vi "Generate Trajectory for Alignment.vi"(8 "Setpoints":T1={"x setpoint"=-0.39, "y setpoint"=-0.8, "th setpoint"=0.0}, 9 "th":dbl=5.222202292601764, 10 "y":dbl=-5.250819805384862, 11 "x":dbl=0.8562227067038787) -> (2 "Updated Waypoints":cluster{"x":dbl, "y":dbl, "th":dbl}[](array[cluster]), 3 "Trajectory Data Out":T3(array[cluster])=[{"Segment Name"="Linear 0", "Type"=enum."Accel Straight", "Traj Pos Points"=[{"x"=0.8100058273974486, "y"=-3.967975741983552, "th"=5.222202301025391}, {"x"=0.7603878706355013, "y"=-3.830783760791278, "th"=5.0782023010253905}, {"x"=0.7073688364180365, "y"=-3.68418791485404, "th"=4.877149425506592}, {"x"=0.6509487247450543, "y"=-3.5281882041718386, "th"=4.676096549987793}, {"x"=0.5911275356165546, "y"=-3.3627846287446737, "th"=4.475043674468994}, {"x"=0.5279052690325376, "y"=-3.1879771885725448, "th"=4.273990798950195}, {"x"=0.46128192499300325, "y"=-3.0037658836554524, "th"=4.072937923431397}, {"x"=0.39465858095346884, "y"=-2.8195545787383596, "th"=3.8718850479125977}, {"x"=0.32803523691393444, "y"=-2.6353432738212668, "th"=3.6708321723937987}, {"x"=0.26141189287440003, "y"=-2.451131968904174, "th"=3.469779296875}, {"x"=0.198189626290383, "y"=-2.276324528732045, "th"=3.2687264213562015}, {"x"=0.1383684371618834, "y"=-2.1109209533048796, "th"=3.0676735458374025}, {"x"=0.0819483254889012, "y"=-1.954921242622678, "th"=2.8666206703186035}, {"x"=0.02892929127143639, "y"=-1.8083253966854402, "th"=2.6655677947998044}, {"x"=-0.020688665490511016, "y"=-1.671133415493166, "th"=2.4645149192810054}, {"x"=-0.06690554479694102, "y"=-1.5433452990458556, "th"=2.2634620437622064}, {"x"=-0.10972134664785363, "y"=-1.4249610473435088, "th"=2.0624091682434074}, {"x"=-0.14913607104324883, "y"=-1.315980660386126, "th"=1.8613562927246083}, {"x"=-0.18514971798312663, "y"=-1.2164041381737067, "th"=1.6603034172058093}, {"x"=-0.21776228746748705, "y"=-1.1262314807062512, "th"=1.4592505416870103}, {"x"=-0.24697377949633004, "y"=-1.0454626879837594, "th"=1.2581976661682113}, {"x"=-0.27278419406965565, "y"=-0.9740977600062313, "th"=1.0571447906494127}, {"x"=-0.29519353118746383, "y"=-0.9121366967736668, "th"=0.8560919151306141}, {"x"=-0.31420179084975464, "y"=-0.8595794982860661, "th"=0.6550390396118155}, {"x"=-0.329808973056528, "y"=-0.816426164543429, "th"=0.45398616409301695}, {"x"=-0.342015077807784, "y"=-0.7826766955457557, "th"=0.2529332885742184}, {"x"=-0.35082010510352263, "y"=-0.7583310912930461, "th"=0.055585002899170455}, {"x"=-0.3562240549437438, "y"=-0.7433893517853002, "th"=0.002236717224122664}, {"x"=-0.35822692732844763, "y"=-0.737851477022518, "th"=0.002236717224122664}], "Traj Vel Points"=[{"V"=7.294446746788231, "Omega"=-0.0, "V vector"={"y"=-7.056933814139086, "x"=-1.8462498434907955}}, {"V"=7.794446746788231, "Omega"=-7.2, "V vector"={"y"=-7.535671418858484, "x"=-1.991747061129249}}, {"V"=8.294446746788232, "Omega"=-10.052643775939941, "V vector"={"y"=-8.011584634482254, "x"=-2.1476402119148625}}, {"V"=8.794446746788232, "Omega"=-10.052643775939941, "V vector"={"y"=-8.486490625788083, "x"=-2.306896278662117}}, {"V"=9.294446746788232, "Omega"=-10.052643775939941, "V vector"={"y"=-8.960371657345226, "x"=-2.4695100913190724}}, {"V"=9.794446746788232, "Omega"=-10.052643775939941, "V vector"={"y"=-9.433210017677535, "x"=-2.635476396794092}}, {"V"=9.794446746788232, "Omega"=-10.052643775939941, "V vector"={"y"=-9.423903981638178, "x"=-2.6685615639393947}}, {"V"=9.794446746788232, "Omega"=-10.052643775939941, "V vector"={"y"=-9.414481906133277, "x"=-2.701613872254829}}, {"V"=9.794446746788232, "Omega"=-10.052643775939941, "V vector"={"y"=-9.404943907179781, "x"=-2.7346329147570203}}, {"V"=9.294446746788232, "Omega"=-10.052643775939941, "V vector"={"y"=-8.91566678376851, "x"=-2.6263332099505634}}, {"V"=8.794446746788232, "Omega"=-10.052643775939941, "V vector"={"y"=-8.427271425386172, "x"=-2.5146351435076726}}, {"V"=8.294446746788232, "Omega"=-10.052643775939941, "V vector"={"y"=-7.939775651158667, "x"=-2.3995435908884546}}, {"V"=7.794446746788232, "Omega"=-10.052643775939941, "V vector"={"y"=-7.453197256780454, "x"=-2.2810635107418573}}, {"V"=7.294446746788232, "Omega"=-10.052643775939941, "V vector"={"y"=-6.967554014150215, "x"=-2.1591999448009993}}, {"V"=6.794446746788232, "Omega"=-10.052643775939941, "V vector"={"y"=-6.482863671006963, "x"=-2.0339580177769934}}, {"V"=6.294446746788232, "Omega"=-10.052643775939941, "V vector"={"y"=-5.99914395056661, "x"=-1.9053429372511914}}, {"V"=5.794446746788232, "Omega"=-10.052643775939941, "V vector"={"y"=-5.516412551158996, "x"=-1.7733599935659488}}, {"V"=5.294446746788232, "Omega"=-10.052643775939941, "V vector"={"y"=-5.034687145865371, "x"=-1.63801455971383}}, {"V"=4.794446746788232, "Omega"=-10.052643775939941, "V vector"={"y"=-4.553985382156366, "x"=-1.4993120912253046}}, {"V"=4.294446746788232, "Omega"=-10.052643775939941, "V vector"={"y"=-4.074324881530425, "x"=-1.3572581260549188}}, {"V"=3.794446746788232, "Omega"=-10.052643775939941, "V vector"={"y"=-3.595723239152738, "x"=-1.2118582844659433}}, {"V"=3.294446746788232, "Omega"=-10.052643775939941, "V vector"={"y"=-3.118198023494648, "x"=-1.0631182689134988}}, {"V"=2.794446746788232, "Omega"=-10.052643775939941, "V vector"={"y"=-2.641766775973572, "x"=-0.9110438639261721}}, {"V"=2.294446746788232, "Omega"=-10.052643775939941, "V vector"={"y"=-2.166447010593411, "x"=-0.7556409359861169}}, {"V"=1.794446746788232, "Omega"=-10.052643775939941, "V vector"={"y"=-1.692256213585474, "x"=-0.5969154334076338}}, {"V"=1.294446746788232, "Omega"=-10.052643775939941, "V vector"={"y"=-1.2192118430499221, "x"=-0.4348733862142511}}, {"V"=0.7944467467882319, "Omega"=-9.867414283752396, "V vector"={"y"=-0.7473487535270189, "x"=-0.26947258503234844}}, {"V"=0.2944467467882319, "Omega"=-2.6674142837523886, "V vector"={"y"=-0.2768976473427397, "x"=-0.1001328097589842}}, {"V"=0.0, "Omega"=-0.0, "V vector"={"y"=-0.0, "x"=-0.0}}], "Accel Index"=6, "Decel Index"=9}, {"Segment Name"="", "Type"=enum."Accel Straight", "Traj Pos Points"=[], "Traj Vel Points"=[], "Accel Index"=0, "Decel Index"=0}])   [LabVIEW 2023]
uses:
  bordeaux-pathinator/Bordeaux/Types/Segment Type.ctl
  bordeaux-pathinator/Bordeaux/Types/Angluar Limits.ctl
  bordeaux-pathinator/Bordeaux/Types/Drive Type.ctl
  bordeaux-pathinator/Bordeaux/Types/Limits.ctl
  Framework/Robot Global Data.vi
panel:
  in  "Ft per ft/sec":dbl=0.167
  out "Expected Distance":dbl=3.664199722009253
  out "Time & Dist":cluster{"Time (s)":dbl, "Distance (ft)":dbl}={"Time (s)"=0.58, "Distance (ft)"=3.664199722009253}
  out "past gen speed":u32=4
  out "Waveform Chart":dbl[](graph)=[7.294446746788231, 7.794446746788231, 8.294446746788232, 8.794446746788232, 9.294446746788232, 9.794446746788232, 9.794446746788232, 9.794446746788232, 9.794446746788232, 9.294446746788232, 8.794446746788232, 8.294446746788232, 7.794446746788232, 7.294446746788232, 6.794446746788232, 6.294446746788232, 5.794446746788232, 5.294446746788232, 4.794446746788232, 4.294446746788232, 3.794446746788232, 3.294446746788232, 2.794446746788232, 2.294446746788232, 1.794446746788232, 1.294446746788232, 0.7944467467882319, 0.2944467467882319, 0.0]
  out "Error":cluster{dbl, dbl, "th":dbl}={1.2462227067038787, -3.4457638584308623, "th"=5.222202292601764}
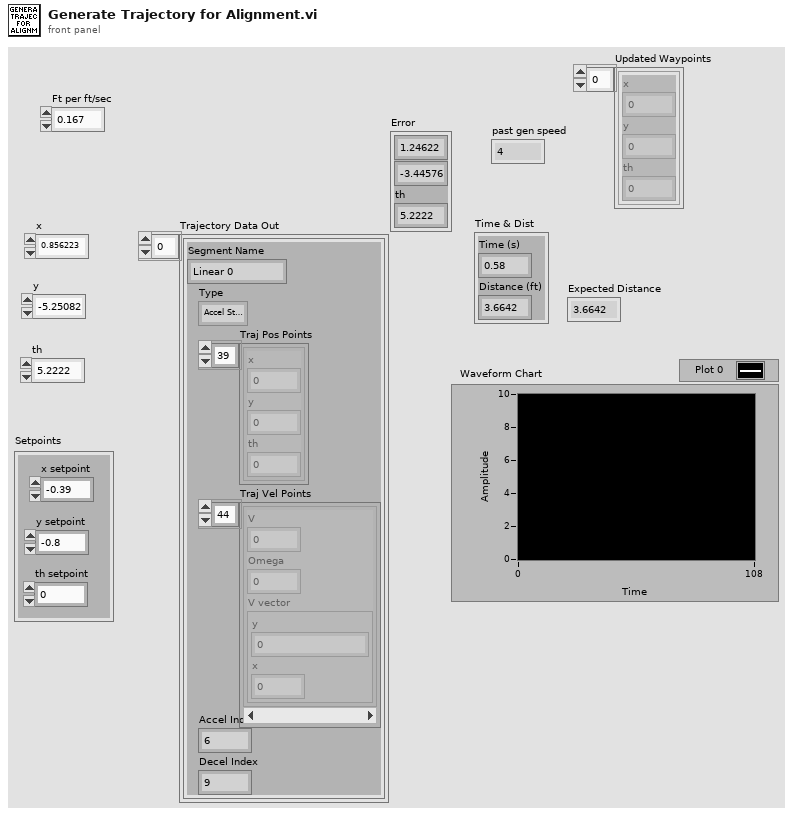
[diagram p1: front panel]
types:
  T1 = cluster{"x setpoint":dbl, "y setpoint":dbl, "th setpoint":dbl}
  T2 = typedef "Segment Type.ctl" = enum16{"Accel Straight", "Const Straight", "Blend", "Circle", "Bezier"}
  T3 = cluster{"Segment Name":string, "Type":T2, "Traj Pos Points":cluster{"x":dbl, "y":dbl, "th":dbl}[], "Traj Vel Points":cluster{"V":dbl, "Omega":dbl, "V vector":cluster{"y":dbl, "x":dbl}}[], "Accel Index":i32, "Decel Index":i32}[]
  T4 = typedef "Limits.ctl" = cluster{"Velocity (fps)":dbl, "Accel (fps^2)":dbl, "Jerk (fps^3)":dbl, "StoopidFast (fps)":dbl}
  T5 = typedef "Drive Type.ctl" = enum16{"Nonholonomic", "Holonomic"}
  T6 = typedef "Angluar Limits.ctl" = cluster{"Velocity (deg/s)":dbl, "Accel (deg/s^2)":dbl, "Jerk (deg/s^3)":dbl}
  T7 = typedef "Robot Velocities.ctl" = cluster{"X Velocity":dbl, "Y Velocity":dbl, "Rotational \nVelocity":dbl}
  T8 = cluster{"x setpoint":dbl, "y setpoint":dbl, "th setpoint":dbl}[]
  T9 = cluster{"V":dbl, "Omega":dbl, "V vector":cluster{"y":dbl, "x":dbl}}[]
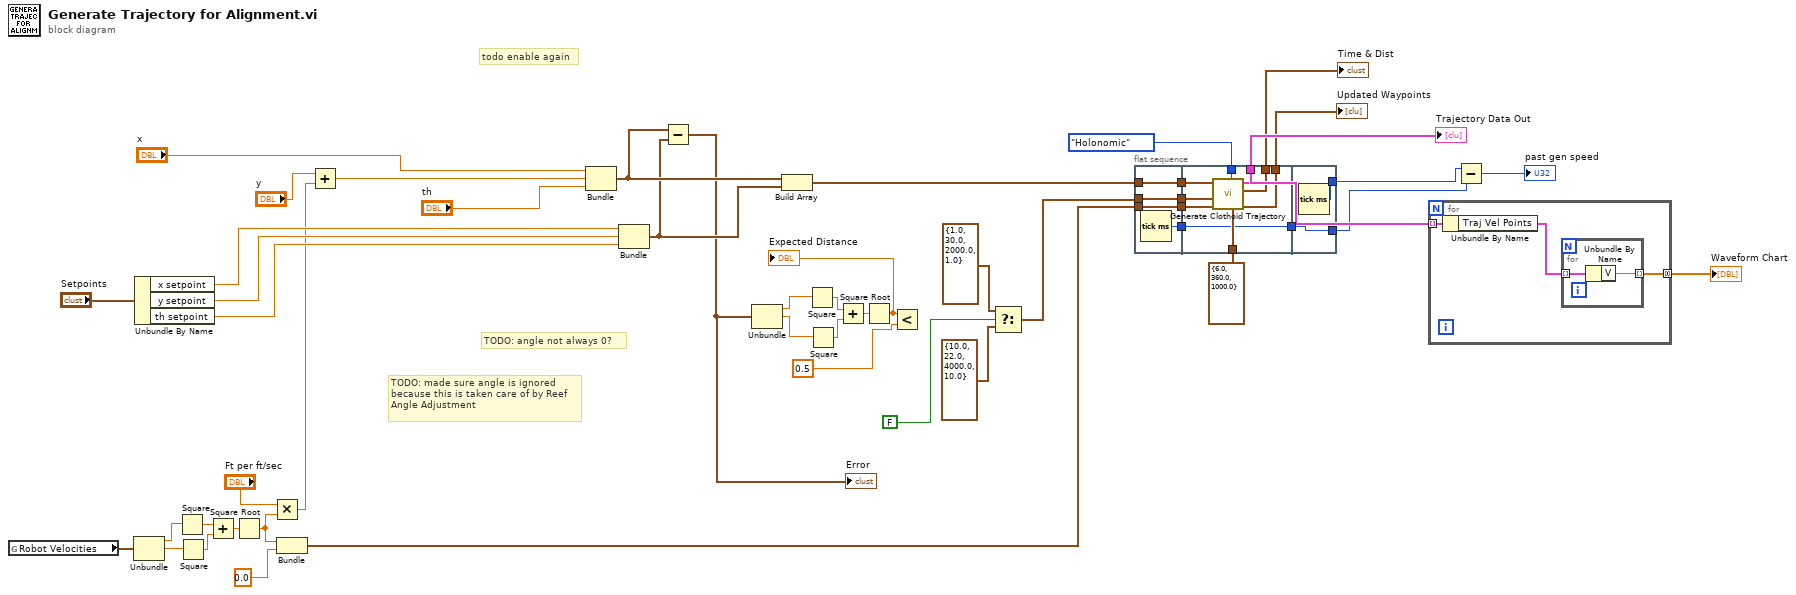
[diagram p0: block diagram]
diagram:
  # "TODO: made sure angle is ignored\nbecause this is taken care of by Reef\nAngle Adjustment"
  # "todo enable again"
  # "TODO: angle not always 0?"
  n1 = global read "Robot Global Data.vi" "Robot Velocities"() -> (w27:T7)
  n2 = Unbundle(w27) -> ("X Velocity"=w22:dbl, "Y Velocity"=w21:dbl)  [unwired: 1 out]
  n3 = Unbundle By Name("Setpoints") -> ("x setpoint"=w45:dbl, "y setpoint"=w44:dbl, "th setpoint"=w30:dbl)
  n4 = Square(x=w22) -> (x^2=w24:dbl)
  n5 = Square(x=w21) -> (x^2=w23:dbl)
  n6 = Add(x=w24, y=w23) -> (x+y=w25:dbl)
  n7 = Square Root(x=w25) -> (sqrt(x)=w7:dbl)
  n8 = Multiply(x="Ft per ft/sec", y=w7) -> (x*y=w4:dbl)
  n9 = Bundle(w7, 0.0) -> (w26:cluster{dbl, dbl})  [unwired: 1 in]
  n10 = Add(x="y", y=w4) -> (x+y=w3:dbl)
  n11 = Bundle("x"="x", w3, "th"="th") -> (w42:cluster{"x":dbl, dbl, "th":dbl})  [unwired: 1 in]
  n12 = Bundle("x setpoint"=w45, "y setpoint"=w44, "th setpoint"=w30) -> (w41:T1)  [unwired: 1 in]
  n13 = Subtract(x=w42, y=w41) -> (x-y=w40:cluster{dbl, dbl, dbl})
  "Error" <- w40
  n14 = Unbundle(w40) -> (w39:dbl, w38:dbl)  [unwired: 1 out]
  n15 = Build Array(w42, w41) -> (w43:T8)
  n16 = Square(x=w39) -> (x^2=w36:dbl)
  n17 = Square(x=w38) -> (x^2=w35:dbl)
  n18 = Add(x=w36, y=w35) -> (x+y=w37:dbl)
  n19 = Square Root(x=w37) -> (sqrt(x)=w8:dbl)
  "Expected Distance" <- w8
  n20 = Less?(x=w8, y=0.5) -> ()  [unwired: 1 out]
  n21 = Select(t=T4 {"Velocity (fps)"=1.0, "Accel (fps^2)"=30.0, "Jerk (fps^3)"=2000.0, "StoopidFast (fps)"=1.0} ("Limits"), s=FALSE, f=T4 {"Velocity (fps)"=10.0, "Accel (fps^2)"=22.0, "Jerk (fps^3)"=4000.0, "StoopidFast (fps)"=10.0} ("Limits")) -> (s? t:f=w32:T4)
  n22 = flat-sequence {
    tunnel: w26 -> [w50]
    tunnel: w32 -> [w51]
    tunnel: w43 -> [w52]
    tunnel: [w52] -> w17
    tunnel: [w51] -> w16
    tunnel: [w50] -> w15
    tunnel: [w49] -> w13
    tunnel: Drive_Type."Holonomic" ("Drive Type") -> [w61]
    tunnel: T6 {"Velocity (deg/s)"=6.0, "Accel (deg/s^2)"=360.0, "Jerk (deg/s^3)"=1000.0} ("Angular Limits") -> [w60]
    tunnel: [w56] -> w19
    tunnel: w17 -> [w59]
    tunnel: w16 -> [w58]
    tunnel: w15 -> [w57]
    tunnel: w13 -> [w55]
    tunnel: [w55] -> w12
    tunnel: [w54] -> w9
    tunnel: [w53] -> w1
    tunnel: [w63] -> w14
    tunnel: w12 -> [w62]
    tunnel: [w62] -> w11
    frame #0 {
      n23 = Tick Count (ms)() -> (millisecond timer value=w49:u32)
    }
    frame #1 {
      n24 = call "Generate Clothoid Trajectory.vi"("Angular Limits"=w60, "Drive Type"=w61, "Conditions"=w57, "Limits"=w58, "WayPoints"=w59) -> ("Updated Waypoints"=w53:cluster{"x":dbl, "y":dbl, "th":dbl}[], "Time & Dist"=w54:cluster{"Time (s)":dbl, "Distance (ft)":dbl}, "Trajectory Data Out"=w56:T3)  [unwired: 3 in, 1 out]
    }
    frame #2 {
      n25 = Tick Count (ms)() -> (millisecond timer value=w63:u32)
    }
  }
  n26 = for {
    tunnel: w19 -> [w66] mode=indexing
    tunnel: [w64] -> w18 mode=concatenating
    n27 = Unbundle By Name(w66) -> ("Traj Vel Points"=w65:T9)
    n28 = for {
      tunnel: w65 -> [w68] mode=indexing
      tunnel: [w67] -> w64 mode=indexing
      n29 = Unbundle By Name(w68) -> ("V"=w67:dbl)
    }
  }
  "Waveform Chart" <- w18
  n30 = Subtract(x=w14, y=w11) -> (x-y=→"past gen speed":u32)
  "Trajectory Data Out" <- w19
  "Time & Dist" <- w9
  "Updated Waypoints" <- w1
